vi "create_target.vi"(11 "Inputs":dbl[](array[numeric])) -> (3 "Target Array":dbl[](array[numeric]))   [LabVIEW 2015]
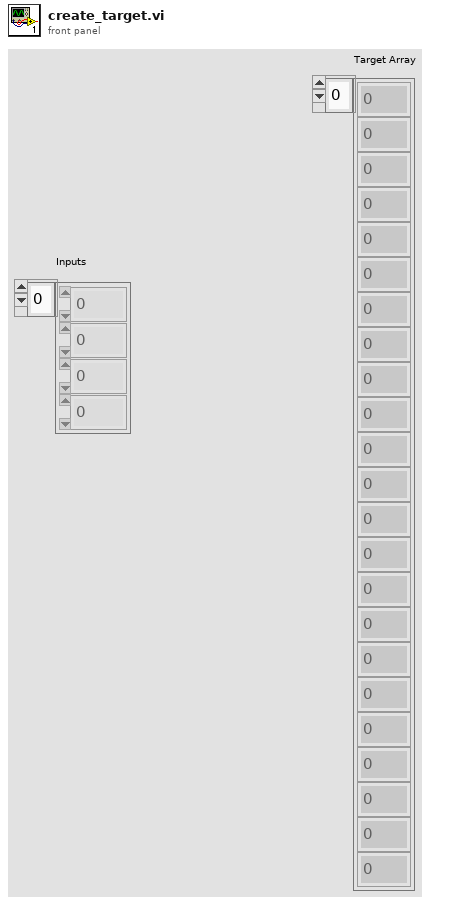
[diagram p1: front panel]
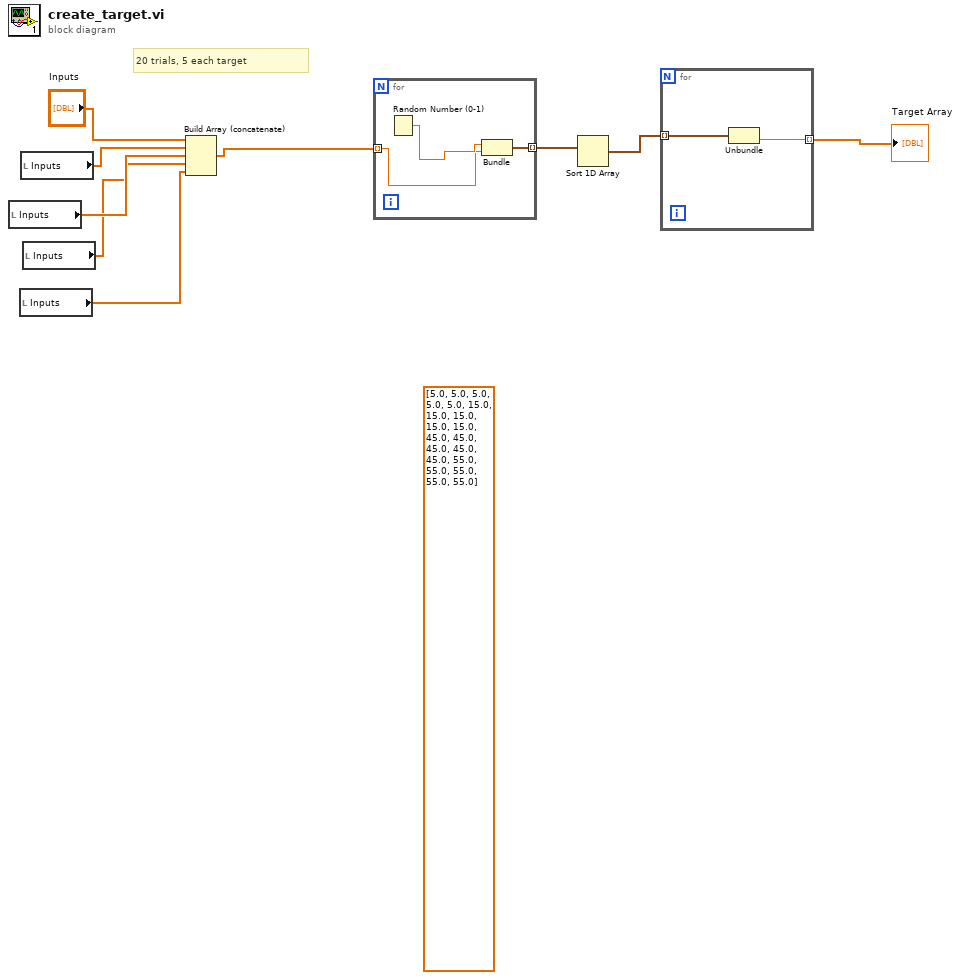
[diagram p0: block diagram]
diagram:
  (unwired) dbl[] [5.0, 5.0, 5.0, 5.0, 5.0, 15.0, 15.0, 15.0, 15.0, 15.0, 45.0, 45.0, 45.0, 45.0, 45.0, 55.0, 55.0, 55.0, 55.0, 55.0]
  # "20 trials, 5 each target"
  n1 = local read "Inputs"() -> (w4:dbl[])
  n2 = local read "Inputs"() -> (w2:dbl[])
  n3 = local read "Inputs"() -> (w5:dbl[])
  n4 = local read "Inputs"() -> (w3:dbl[])
  n5 = Build Array (concatenate)("Inputs", w5, w4, w3, w2) -> (w1:dbl[])
  n6 = for {
    tunnel: w1 -> [w11] mode=indexing
    tunnel: [w10] -> w8 mode=indexing
    n7 = Random Number (0-1)() -> (number: 0 to 1=w12:dbl)
    n8 = Bundle("number: 0 to 1"=w12, "Numeric"=w11) -> (w10:cluster{"number: 0 to 1":dbl, "Numeric":dbl})  [unwired: 1 in]
  }
  n9 = Sort 1D Array(array=w8) -> (sorted array=w9:cluster{"number: 0 to 1":dbl, "Numeric":dbl}[])
  n10 = for {
    tunnel: w9 -> [w14] mode=indexing
    tunnel: [w13] -> w7 mode=indexing
    n11 = Unbundle(w14) -> ("Numeric"=w13:dbl)  [unwired: 1 out]
  }
  "Target Array" <- w7
